vi "USB2XXX_LINEX_MasterSchTest.vi"() -> ()   [LabVIEW 2010]
uses:
  PublicFiles/USB2XXX.dll
panel:
  in  "Get Sch":bool
  out "设置调度表成功？":bool
  in  "pInMsg 3":T1={"Timestamp"=50, "MsgType"=2, "CheckType"=0, "DataLen"=0, "Sync"=85, "PID"=3, "Data[0]"=0, "Data[1]"=0, "Data[2]"=0, "Data[3]"=0, "Data[4]"=0, "Data[5]"=0, "Data[6]"=0, "Data[7]"=0, "Check"=0, "Reserve"=0, "Reserve"=0} {"Sync" format="%x"; "PID" format="%x"; "Data[0]" format="%x"; "Data[1]" format="%x"; "Data[2]" format="%x"; "Data[3]" format="%x"; "Data[4]" format="%x"; "Data[5]" format="%x"; "Data[6]" format="%x"; "Data[7]" format="%x"; "Check" format="%x"; "Reserve" format="%x"; "Reserve" format="%x"}
  in  "pInMsg 2":T1={"Timestamp"=50, "MsgType"=1, "CheckType"=0, "DataLen"=8, "Sync"=85, "PID"=2, "Data[0]"=17, "Data[1]"=34, "Data[2]"=51, "Data[3]"=68, "Data[4]"=85, "Data[5]"=102, "Data[6]"=119, "Data[7]"=136, "Check"=0, "Reserve"=0, "Reserve"=0} {"Sync" format="%x"; "PID" format="%x"; "Data[0]" format="%x"; "Data[1]" format="%x"; "Data[2]" format="%x"; "Data[3]" format="%x"; "Data[4]" format="%x"; "Data[5]" format="%x"; "Data[6]" format="%x"; "Data[7]" format="%x"; "Check" format="%x"; "Reserve" format="%x"; "Reserve" format="%x"}
  out "pOutMsg":T2(array[cluster]) {"Sync" format="%x"; "PID" format="%x"; "Data[0]" format="%x"; "Data[1]" format="%x"; "Data[2]" format="%x"; "Data[3]" format="%x"; "Data[4]" format="%x"; "Data[5]" format="%x"; "Data[6]" format="%x"; "Data[7]" format="%x"; "Check" format="%x"}
  in  "pInMsg":T1={"Timestamp"=50, "MsgType"=1, "CheckType"=0, "DataLen"=8, "Sync"=85, "PID"=1, "Data[0]"=1, "Data[1]"=2, "Data[2]"=3, "Data[3]"=4, "Data[4]"=5, "Data[5]"=6, "Data[6]"=7, "Data[7]"=8, "Check"=0, "Reserve"=0, "Reserve"=0} {"Sync" format="%x"; "PID" format="%x"; "Data[0]" format="%x"; "Data[1]" format="%x"; "Data[2]" format="%x"; "Data[3]" format="%x"; "Data[4]" format="%x"; "Data[5]" format="%x"; "Data[6]" format="%x"; "Data[7]" format="%x"; "Check" format="%x"; "Reserve" format="%x"; "Reserve" format="%x"}
  out "function return":i32
  in  "BaudRate":u32=9600
  in  "Channel Index":u8(ring) items=["CH0"]
  in  "Device Index":i32(ring) items=["0", "1", "2", "3", "4", "5"]
  out "Flag(T:Write;F:Read)":bool=TRUE
  in  "stop":bool
  in  "Read":bool
  in  "Write":bool
  # "波特率一定要设置，否则程序可能出错"
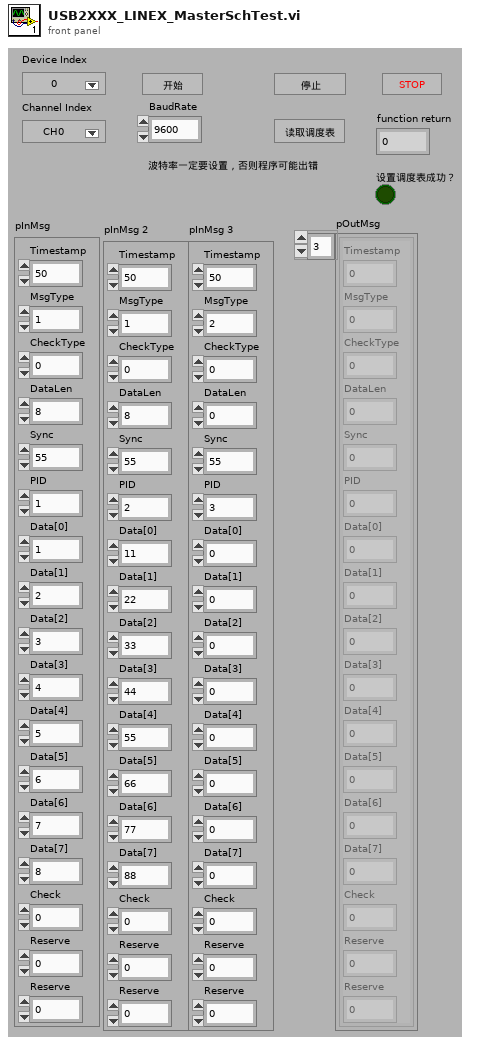
[diagram p1: front panel]
types:
  T1 = cluster{"Timestamp":u32, "MsgType":u8, "CheckType":u8, "DataLen":u8, "Sync":u8, "PID":u8, "Data[0]":u8, "Data[1]":u8, "Data[2]":u8, "Data[3]":u8, "Data[4]":u8, "Data[5]":u8, "Data[6]":u8, "Data[7]":u8, "Check":u8, "Reserve":u8, "Reserve":u8}
  T2 = cluster{"Timestamp":u32, "MsgType":u8, "CheckType":u8, "DataLen":u8, "Sync":u8, "PID":u8, "Data[0]":u8, "Data[1]":u8, "Data[2]":u8, "Data[3]":u8, "Data[4]":u8, "Data[5]":u8, "Data[6]":u8, "Data[7]":u8, "Check":u8, "Reserve":u8, "Reserve":u8}[]
  T3 = enum16{"Init", "Write", "Read", "Idel", "Close", "GetSch"}
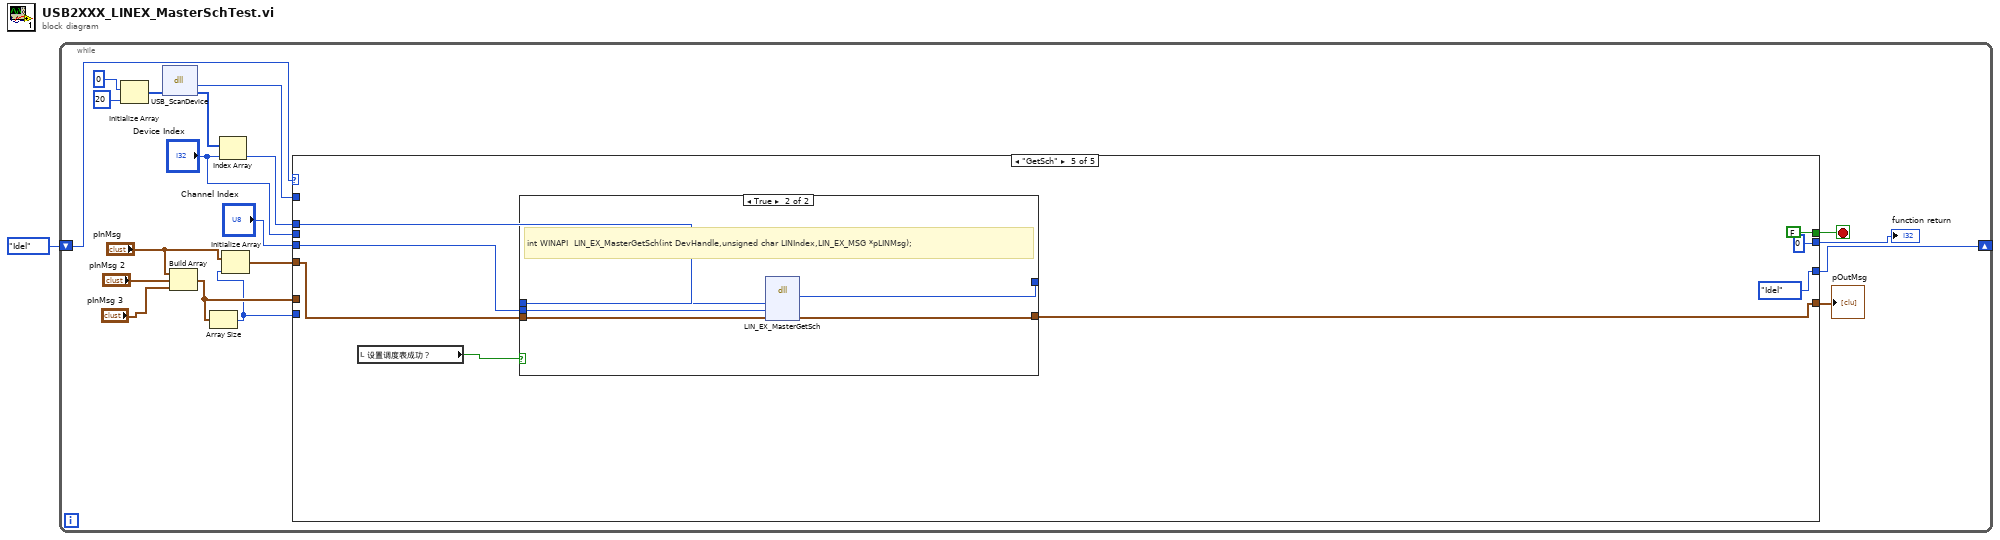
[diagram p0: block diagram]
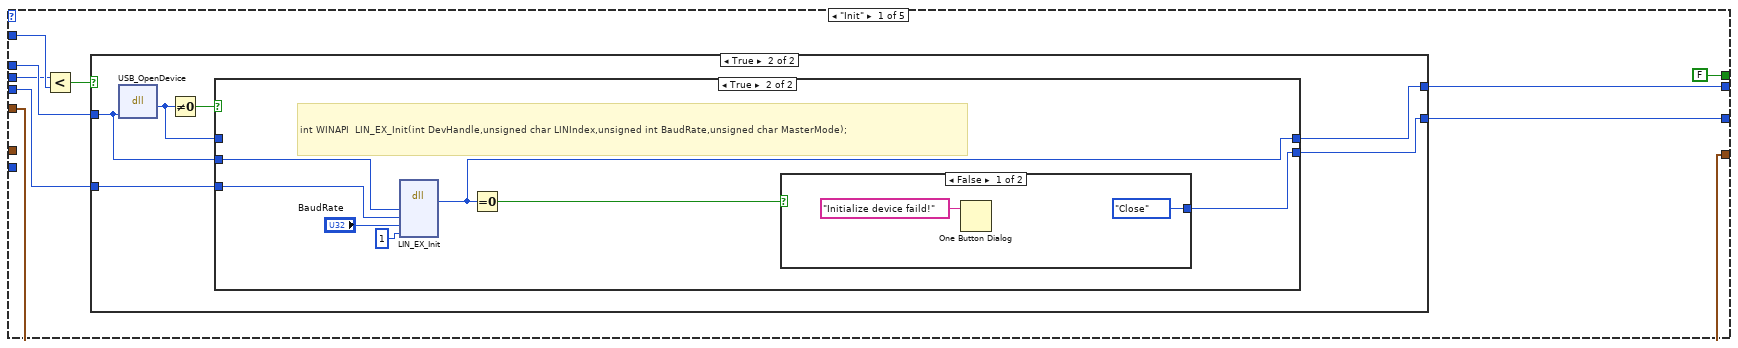
[diagram p2: hidden frame]
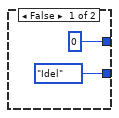
[diagram p3: hidden frame]
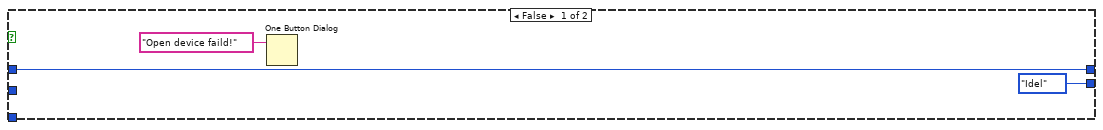
[diagram p4: hidden frame]
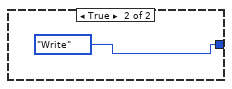
[diagram p5: hidden frame]
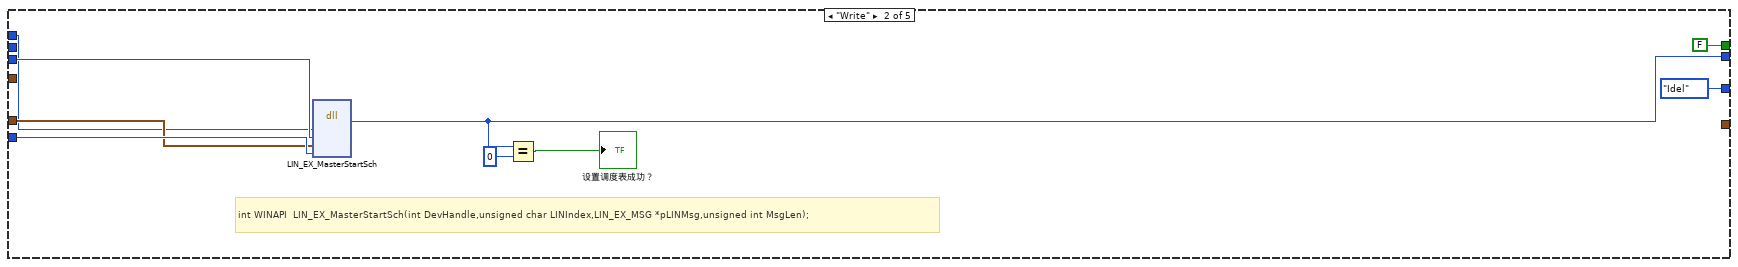
[diagram p6: hidden frame]
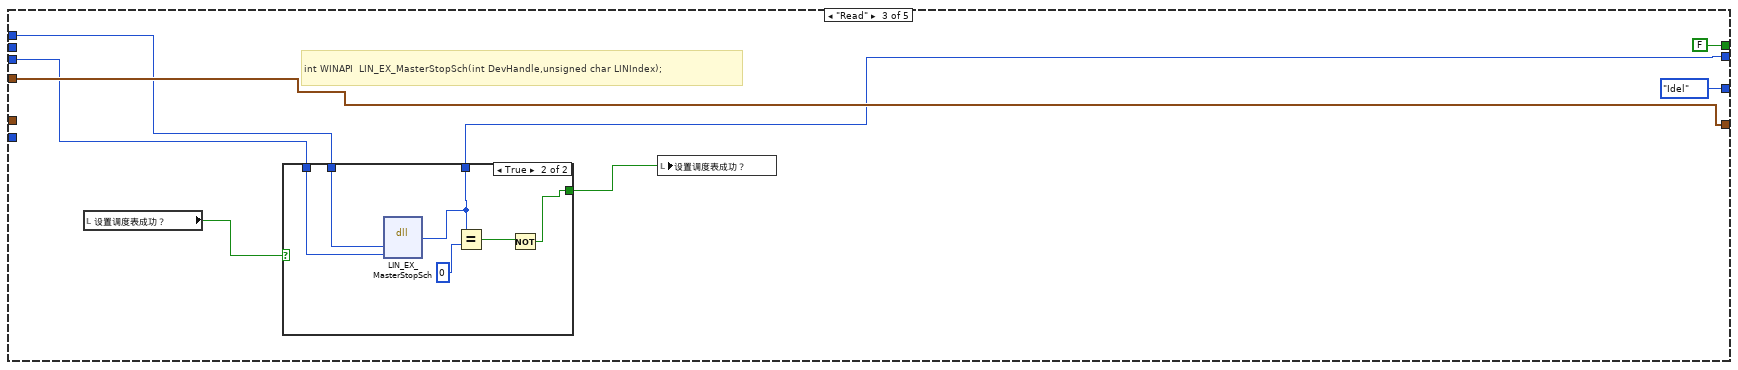
[diagram p7: hidden frame]
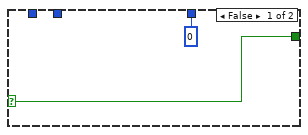
[diagram p8: hidden frame]
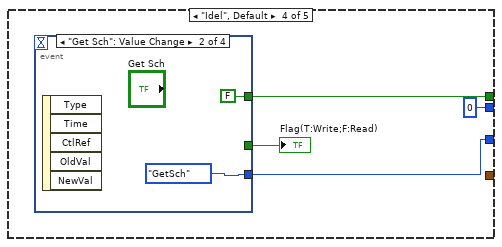
[diagram p9: hidden frame]
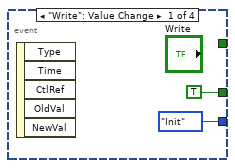
[diagram p10: hidden frame]
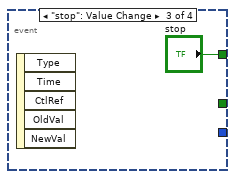
[diagram p11: hidden frame]
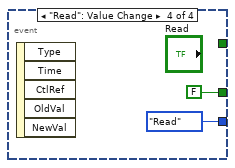
[diagram p12: hidden frame]
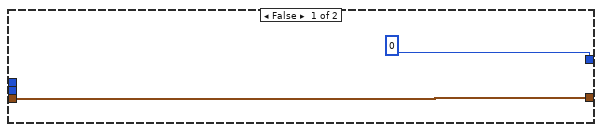
[diagram p13: hidden frame]
diagram:
  n1 = while {
    shift-right: [w19] -> _
    shift-left: T3."Idel" ("Enum") -> [w20]
    stop <- w17 stop-if-true
    n2 = Initialize Array(0, 20 ("dimension size")) -> (w16:i32[])
    n3 = dll-call lib="E:/OtherWork/STM32/USB2XXX_Example/trunk/Labview/PublicFiles/USB2XXX.dll" fn="USB_ScanDevice"("pDevNum"=w16) -> ("return type"=w12:i32, "pDevNum"=w13:i32[])  [unwired: 3 in, 2 out]
    n4 = Build Array("pInMsg", "pInMsg 2", "pInMsg 3") -> (w3:T2)
    n5 = Array Size(array=w3) -> (size(s)=w2:i32)
    n6 = Index Array(array=w13, index="Device Index") -> (element=w7:i32)
    n7 = Initialize Array("pInMsg", w2) -> (w10:T2)
    n8 = case shown="\"GetSch\"" w20 {
      tunnel: [w28 T3."Idel" ("Enum") T3."Idel" ("Enum") w77 T3."Idel" ("Enum")] -> w19
      tunnel: w7 -> [w24 w54 w62 _ w91]
      tunnel: "Channel Index" -> [w27 w55 w61 _ w90]
      tunnel: [FALSE FALSE FALSE w78 FALSE] -> w17
      tunnel: w12 -> [w25 _ _ _ _]
      tunnel: "Device Index" -> [w23 _ _ _ _]
      tunnel: w2 -> [_ w57 _ _ _]
      tunnel: w10 -> [w22 _ w65 _ w89]
      tunnel: w3 -> [_ w56 _ _ _]
      tunnel: [w22 _ w65 _ w88] -> w9
      tunnel: [w21 w53 w64 0 ("return type") 0 ("return type")] -> w8
      frame "Init" {
        n9 = Less?(x=w23, y=w25) -> (x < y?=w29:bool)
        n10 = case shown="True" w29 {
          tunnel: w24 -> [_ w35]
          tunnel: w27 -> [_ w36]
          tunnel: [T3."Idel" ("Enum") w34] -> w28
          tunnel: [0 ("return type") w33] -> w21
          frame False {
          }
          frame True {
            n11 = dll-call lib="E:/OtherWork/STM32/USB2XXX_Example/trunk/Labview/PublicFiles/USB2XXX.dll" fn="USB_OpenDevice"("DevIndex"=w35) -> ("return type"=w32:u8)  [unwired: 4 in, 2 out]
            n12 = Not Equal To 0?(x=w32) -> (x != 0?=w37:bool)
            n13 = case shown="True" w37 {
              tunnel: w36 -> [_ w43]
              tunnel: w35 -> [_ w44]
              tunnel: [T3."Idel" ("Enum") w46] -> w34
              tunnel: [w38 w41] -> w33
              tunnel: w32 -> [w38 _]
              frame False {
                n14 = One Button Dialog(message="Open device faild!") -> ()  [unwired: 1 in, 1 out]
              }
              frame True {
                # "int WINAPI  LIN_EX_Init(int DevHandle,unsigned char LINIndex,unsigned int BaudRate,unsigned char MasterMode);"
                n15 = dll-call lib="E:/OtherWork/STM32/USB2XXX_Example/trunk/Labview/PublicFiles/USB2XXX.dll" fn="LIN_EX_Init"("DevHandle"=w44, "LINIndex"=w43, "BaudRate"="BaudRate", "MasterMode"=u8 1) -> ("return type"=w41:i32)  [unwired: 7 in, 2 out]
                n16 = Equal To 0?(x=w41) -> (x = 0?=w47:bool)
                n17 = case shown="False" w47 {
                  tunnel: [T3."Close" ("Enum") T3."Write" ("Enum")] -> w46
                  frame False {
                    n18 = One Button Dialog(message="Initialize device faild!") -> ()  [unwired: 1 in, 1 out]
                  }
                  frame True {
                  }
                }
              }
            }
          }
        }
      }
      frame "Write" {
        # "int WINAPI  LIN_EX_MasterStartSch(int DevHandle,unsigned char LINIndex,LIN_EX_MSG *pLINMsg,unsigned int MsgLen);"
        n19 = dll-call lib="E:/OtherWork/STM32/USB2XXX_Example/trunk/Labview/PublicFiles/USB2XXX.*" fn="LIN_EX_MasterStartSch"("DevHandle"=w54, "LINIndex"=w55, "pLINMsg"=w56, "MsgLen"=w57) -> ("return type"=w53:i32)  [unwired: 7 in, 2 out]
        n20 = Equal?(x=w53, y=0) -> (x = y?=→"设置调度表成功？":bool)
      }
      frame "Read" {
        # "int WINAPI  LIN_EX_MasterStopSch(int DevHandle,unsigned char LINIndex);"
        n21 = local read "设置调度表成功？"() -> (w63:bool)
        n22 = case shown="True" w63 {
          selector: w63 -> [w68 _]
          tunnel: [0 w72] -> w64
          tunnel: [w68 w70] -> w60
          tunnel: w62 -> [_ w74]
          tunnel: w61 -> [_ w73]
          frame False {
          }
          frame True {
            n23 = dll-call lib="E:/OtherWork/STM32/USB2XXX_Example/trunk/Labview/PublicFiles/USB2XXX.*" fn="LIN_EX_MasterStopSch"("DevHandle"=w74, "LINIndex"=w73) -> (w72:i32)  [unwired: 5 in, 2 out]
            n24 = Equal?(x=w72, y=0) -> (x = y?=w71:bool)
            n25 = Not(x=w71) -> (.not. x?=w70:bool)
          }
        }
        n26 = local write "设置调度表成功？"(w60) -> ()
      }
      frame "Idel", Default {
        n27 = event shown="[1] \"Get Sch\": Value Change" {
          selector: _ -> [_ _ _ _]
          dyn-events: _ -> [_ _ _ _]
          timeout: _ -> [_ _ _ _]
          tunnel: [TRUE _ _ FALSE] -> w79
          tunnel: [_ FALSE ("stop") "stop" _] -> w78
          tunnel: [T3."Init" ("Enum") T3."GetSch" ("Enum") _ T3."Read" ("Enum")] -> w77
          event "Write": Value Change {
            n28 = event-data() -> ()  [unwired: 1 in, 5 out]
          }
          event "Get Sch": Value Change {
            n29 = event-data() -> ()  [unwired: 1 in, 5 out]
          }
          event "stop": Value Change {
            n30 = event-data() -> ()  [unwired: 1 in, 5 out]
          }
          event "Read": Value Change {
            n31 = event-data() -> ()  [unwired: 1 in, 5 out]
          }
        }
        "Flag(T:Write;F:Read)" <- w79
      }
      frame "GetSch" {
        n32 = local read "设置调度表成功？"() -> (w92:bool)
        n33 = case shown="True" w92 {
          tunnel: w91 -> [_ w101]
          tunnel: w90 -> [_ w100]
          tunnel: w89 -> [w96 w99]
          tunnel: [0 w98] -> _
          tunnel: [w96 w97] -> w88
          frame False {
          }
          frame True {
            # "int WINAPI  LIN_EX_MasterGetSch(int DevHandle,unsigned char LINIndex,LIN_EX_MSG *pLINMsg);"
            n34 = dll-call lib="E:/OtherWork/STM32/USB2XXX_Example/trunk/Labview/PublicFiles/USB2XXX.*" fn="LIN_EX_MasterGetSch"("DevHandle"=w101, "LINIndex"=w100, "pLINMsg"=w99) -> ("return type"=w98:i32, "pLINMsg"=w97:T2)  [unwired: 5 in, 2 out]
          }
        }
      }
    }
    "pOutMsg" <- w9
    "function return" <- w8
  }
